vi "Vstep2VBoard.vi"(8 "Axis":dbl, 11 "Speed (usteps/sec)":dbl) -> (3 "Maximum Positioning Speed (Board Units)":dbl)   [LabVIEW 2013]
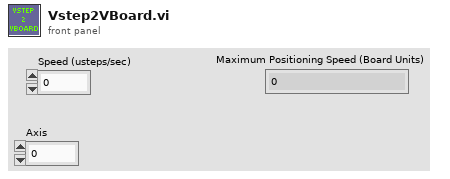
[diagram p1: front panel]
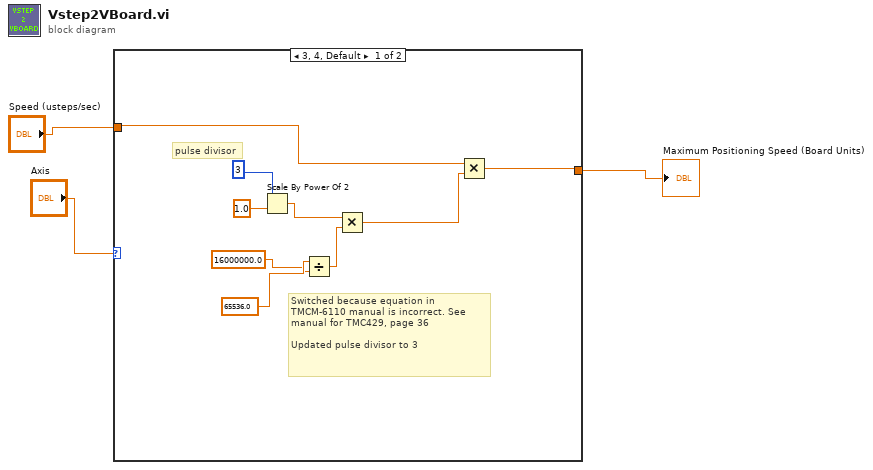
[diagram p0: block diagram]
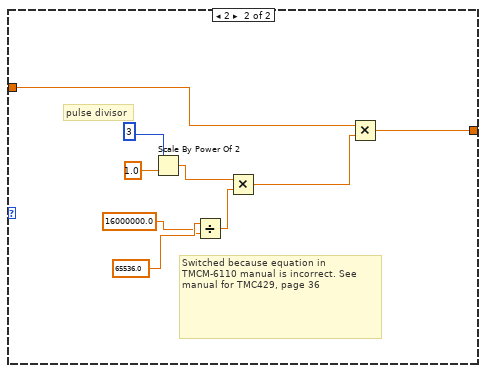
[diagram p2: hidden frame]
diagram:
  n1 = case shown="3, 4, Default" "Axis" {
    tunnel: [w4 w16] -> w3
    tunnel: "Speed (usteps/sec)" -> [w5 w13]
    frame 3, 4, Default {
      # "Switched because equation in TMCM-6110 manual is incorrect. See manual for TMC429, page 36\n\nUpdated pulse divisor to 3"
      # "pulse divisor"
      n2 = Scale By Power Of 2(n=i16 3, x=1.0) -> (x*2^n=w9:dbl)
      n3 = Divide(x=65536.0 ("y"), y=16000000.0 ("x")) -> (x/y=w12:dbl)
      n4 = Multiply(x=w9, y=w12) -> (x*y=w8:dbl)
      n5 = Multiply(x=w5, y=w8) -> (x*y=w4:dbl)
    }
    frame 2 {
      # "Switched because equation in TMCM-6110 manual is incorrect. See manual for TMC429, page 36"
      # "pulse divisor"
      n6 = Scale By Power Of 2(n=i16 3, x=1.0) -> (x*2^n=w18:dbl)
      n7 = Divide(x=65536.0 ("y"), y=16000000.0 ("x")) -> (x/y=w21:dbl)
      n8 = Multiply(x=w18, y=w21) -> (x*y=w17:dbl)
      n9 = Multiply(x=w13, y=w17) -> (x*y=w16:dbl)
    }
  }
  "Maximum Positioning Speed (Board Units)" <- w3
